vi "PUT Reload Config Event.vi"(0 "Reload Config Event":refnum<user-event>) -> ()   [LabVIEW 2013]
uses:
  Functional Globals/Action.ctl
  Event Selector.ctl
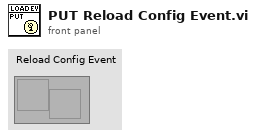
[diagram p1: front panel]
types:
  T1 = typedef "Event Selector.ctl" = enum16{"Stop", "Reload Config"}
  T2 = typedef "Action.ctl" = enum16{"GET", "PUT", "DELETE"}
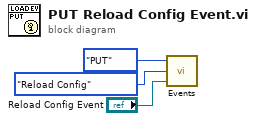
[diagram p0: block diagram]
diagram:
  n1 = call "Events.vi"("Input"="Reload Config Event", "Event Type"=Event_Selector."Reload Config", "Action"=Action."PUT") -> ()  [unwired: 1 out]
